vi "Write User file.vi"(8 "error in":errorcluster, 10 "Array":T1[](array[typedef]), 11 "file path (use dialog)":path) -> (0 "error out":errorcluster, 3 "path":path)   [LabVIEW 2012]
uses:
  typedef/User_Data_Cluster.ctl
  typedef/User Accounts.ctl
panel:
  out "xml string":string
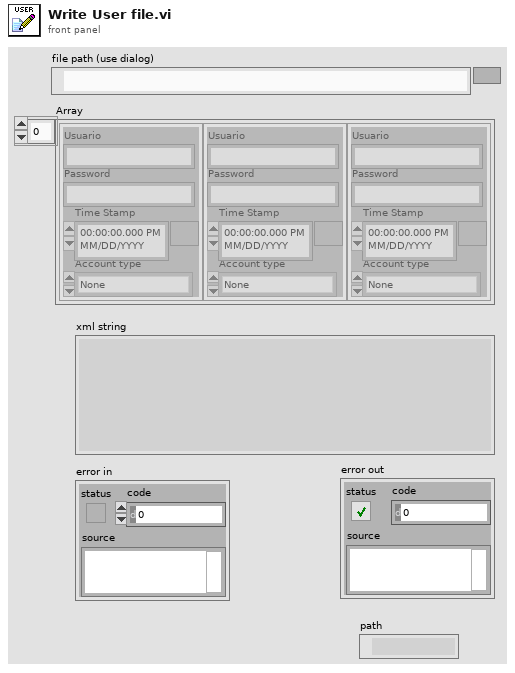
[diagram p1: front panel]
types:
  T1 = typedef "User_Data_Cluster.ctl" = cluster{"Usuario":string, "Password":string, "Account type":T2, "Time Stamp":timestamp}
  T2 = typedef "User Accounts.ctl" = enum16{"None", "User", "Admin"}
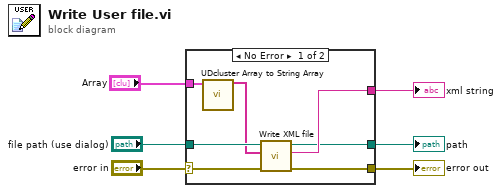
[diagram p0: block diagram]
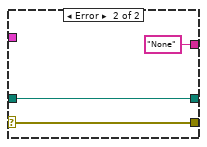
[diagram p2: hidden frame]
diagram:
  n1 = case shown="No Error" "error in" {
    selector: "error in" -> [w9 w16]
    tunnel: "file path (use dialog)" -> [w13 w15]
    tunnel: "Array" -> [w8 _]
    tunnel: [w12 "None" ("xml string")] -> w4
    tunnel: [w11 w16] -> w3
    tunnel: [w10 w15] -> w2
    frame No Error {
      n2 = call "UDcluster Array to String Array.vi"("Array in"=w8) -> ("Array out"=w7:string[])  [unwired: 13 in, 1 out]
      n3 = call "Write XML file.vi"("error in (no error)"=w9, "Array in"=w7, "file path (use dialog)"=w13) -> ("error out"=w11:errorcluster, "xml string"=w12:string, "path"=w10:path)  [unwired: 6 in]
    }
    frame Error {
    }
  }
  "xml string" <- w4
  "error out" <- w3
  "path" <- w2
